vi "Set Calling VI Wnd Top & Active.vi"(8 "Error In":errorcluster) -> (0 "Error Out":errorcluster)   [LabVIEW 2020]
doc: "Sets the Caller VIs front panel Top (other windows can be moved in front), Active (title bar is selected), and gives Focus (keystrokes are directed to the panel).\n\nCopyright © 2010 Blue Ridge Test, Inc.\nwww.BlueRidgeTest.com"
uses:
  USER32.DLL
panel:
  out "Show\\Rest":i32
  out "Minimized?":i32
  out "FG hWnd":i32
  out "FG ProcID":i32
  out "hWnd ProcID":i32
  out "SetFG\\Attach":i32
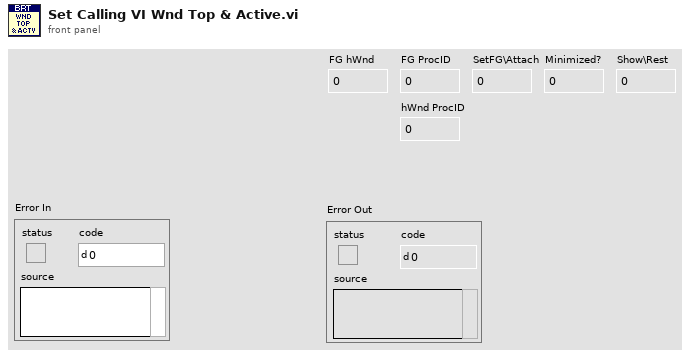
[diagram p1: front panel]
types:
  T1 = enum32{"Invalid", "Standard", "Closed", "Hidden", "Minimized", "Maximized"}
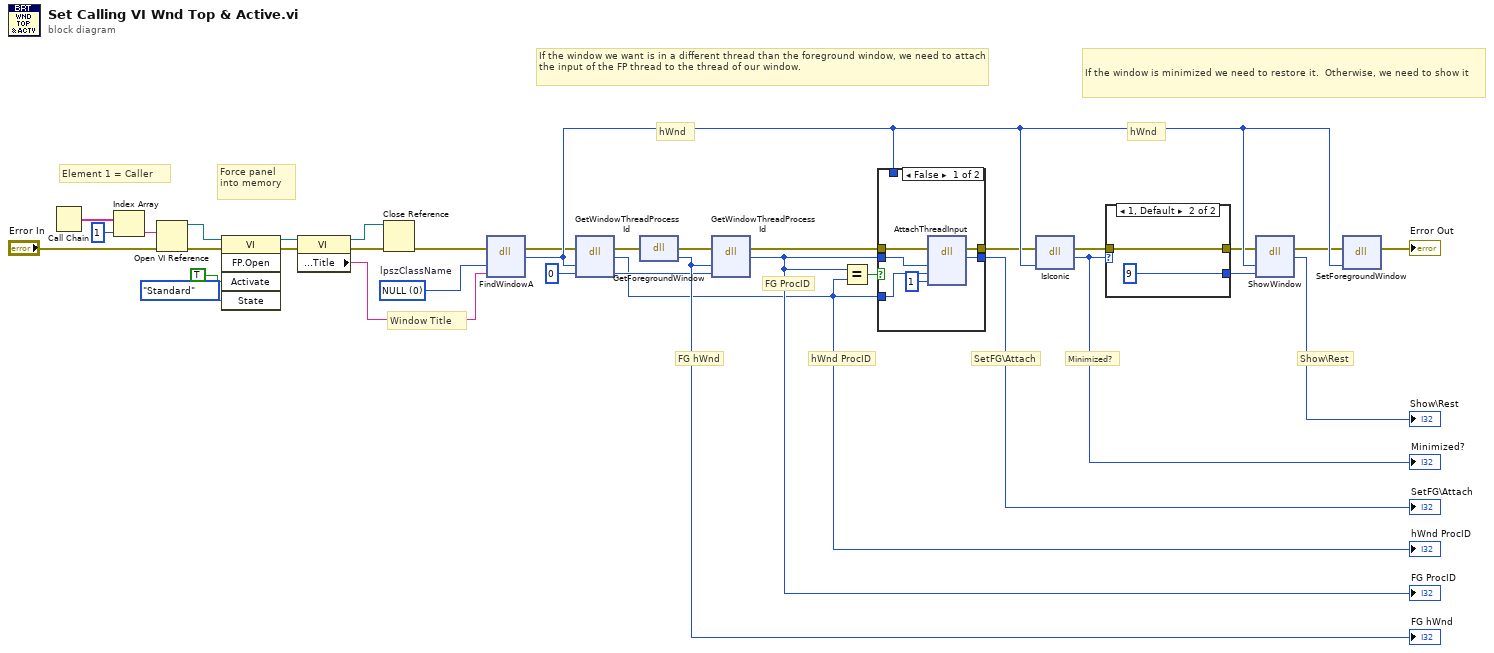
[diagram p0: block diagram]
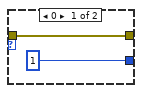
[diagram p2: hidden frame]
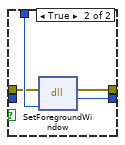
[diagram p3: hidden frame]
diagram:
  w14 = 0 ("lpdwProcessID")
  w32 = 0 items=["NULL"]  # lpszClassName
  # "hWnd ProcID"
  # "Show\\Rest"
  # "Minimized?"
  # "SetFG\\Attach"
  # "Force panel\ninto memory"
  # "FG hWnd"
  # "FG ProcID"
  # "hWnd"
  # "If the window is minimized we need to restore it.  Otherwise, we need to show it"
  # "hWnd"
  # "If the window we want is in a different thread than the foreground window, we need to attach the input of the FP thread to the thread of our window."
  # "Window Title"
  # "Element 1 = Caller"
  n1 = Call Chain() -> (call chain=w30:string[])
  n2 = Index Array(array=w30, index=1) -> (element=w29:string)
  n3 = Open VI Reference(vi path=w29, error in (no error)="Error In") -> (vi reference=w26:refnum<vi>, error out=w27:errorcluster)  [unwired: 4 in]
  n4 = invoke class="VI" method="FP.Open"(reference=w26, error in=w27, "Activate"=TRUE ("Activate?"), "State"=T1."Standard") -> (reference out=w24:refnum<vi>, error out=w25:errorcluster)  [unwired: 1 in, 3 out]
  n5 = property class="VI"(reference=w24, error in=w25) -> (reference out=w22:refnum<vi>, error out=w21:errorcluster, "Front Panel.Title"=w23:string)
  n6 = Close Reference(reference=w22, error in (no error)=w21) -> (error out=w20:errorcluster)
  n7 = dll-call lib="USER32.DLL" fn="FindWindowA" label="FindWindow"(error in=w20, "lpszClassName"=w32, "lpszWindowName"=w23) -> (error out=w16:errorcluster, "hWnd"=w19:u32)  [unwired: 4 in, 1 out]
  n8 = dll-call lib="user32" fn="GetWindowThreadProcessId" label="Get\nWindow\nThread\nProcess\nId"(error in=w16, "hWnd"=w19, "lpdwProcessID"=w14) -> (error out=w9:errorcluster, w8:i32)  [unwired: 4 in, 1 out]
  "hWnd ProcID" <- w8
  n9 = dll-call lib="user32" fn="GetForegroundWindow" label="Get\nForeground\nWindow"(error in=w9) -> (error out=w10:errorcluster, "hWnd"=w15:i32)  [unwired: 2 in, 1 out]
  "FG hWnd" <- w15
  n10 = dll-call lib="user32" fn="GetWindowThreadProcessId" label="Get\nWindow\nThread\nProcess\nId"(error in=w10, "hWnd"=w15, "lpdwProcessID"=w14) -> (error out=w7:errorcluster, w12:i32)  [unwired: 4 in, 1 out]
  "FG ProcID" <- w12
  n11 = Equal?(x=w12, y=w8) -> (x = y?=w13:bool)
  n12 = case shown="False" w13 {
    tunnel: w12 -> [w40 _]
    tunnel: w8 -> [w39 _]
    tunnel: w19 -> [_ w44]
    tunnel: [w37 w43] -> w11
    tunnel: w7 -> [w36 w42]
    tunnel: [w35 w41] -> w18
    frame False {
      n13 = dll-call lib="user32" fn="AttachThreadInput" label="Attach\nThread\nInput"(error in=w36, "idAttach"=w40, "idAttachTo"=w39, "fAttach"=1) -> (error out=w35:errorcluster, w37:i32)  [unwired: 5 in, 1 out]
    }
    frame True {
      n14 = dll-call lib="user32" fn="SetForegroundWindow" label="Set\nForeground\nWindow"(error in=w42, "hWnd"=w44) -> (error out=w41:errorcluster, w43:i32)  [unwired: 3 in, 1 out]
    }
  }
  "SetFG\\Attach" <- w11
  n15 = dll-call lib="user32" fn="IsIconic"(error in=w18, "hWnd"=w19) -> (error out=w2:errorcluster, w6:i32)  [unwired: 3 in, 1 out]
  "Minimized?" <- w6
  n16 = case shown="1, Default" w6 {
    tunnel: [i16 1 ("nCmdshow") i16 9 ("nCmdshow")] -> w5
    tunnel: [w45 w47] -> w3
    tunnel: w2 -> [w45 w47]
    frame 0 {
    }
    frame 1, Default {
    }
  }
  n17 = dll-call lib="user32.dll" fn="ShowWindow"(error in=w3, "hWnd"=w19, "nCmdshow"=w5) -> (error out=w17:errorcluster, →"Show\\Rest":i32)  [unwired: 4 in, 1 out]
  n18 = dll-call lib="user32" fn="SetForegroundWindow" label="Set\nForeground\nWindow"(error in=w17, "hWnd"=w19) -> (error out=→"Error Out":errorcluster)  [unwired: 4 in, 1 out]
